vi "Get Magnet.vi"(6 "Axis":T1, 8 "error in (no error)":errorcluster, 11 "Instrument.Oxford1820 in":refnum<class "Instrument.Oxford1820.lvclass">) -> (0 "error out":errorcluster, 1 "Status":string, 2 "B Field (T)":dbl, 3 "Instrument.Oxford1820 out":refnum<class "Instrument.Oxford1820.lvclass">, 4 "Finished?":bool)   [LabVIEW 2019, in "Instrument.Oxford1820.lvclass"]
uses:
  Instrument.Oxford1820.lvclass
  <userlib>/LevyLab/Instrument Framework/Instrument Types/Cryostat/Typedefs/Magnet Axis--Enum.ctl
  4d514aa9-5884-4ec3-9942-9e0d55515c9c.vi
  Typedefs/Instrument.Oxford1820.Commands-enum.ctl
  c1f1fec1-7ced-457a-8a6a-e70d4f1fe444.vi
  <userlib>/LevyLab/LV-Data/LV-Data.PG/LV-Data.PGSQL.lvclass
  <userlib>/LevyLab/LV-Data/LV-Data.PG/API/Read Variable (string).vi
  <userlib>/LevyLab/LV-Data/LV-Data.PG/API/Read Variable (double).vi
  <userlib>/LevyLab/Instrument Framework/Instrument Types/Cryostat/Instrument.Cryostat.lvclass
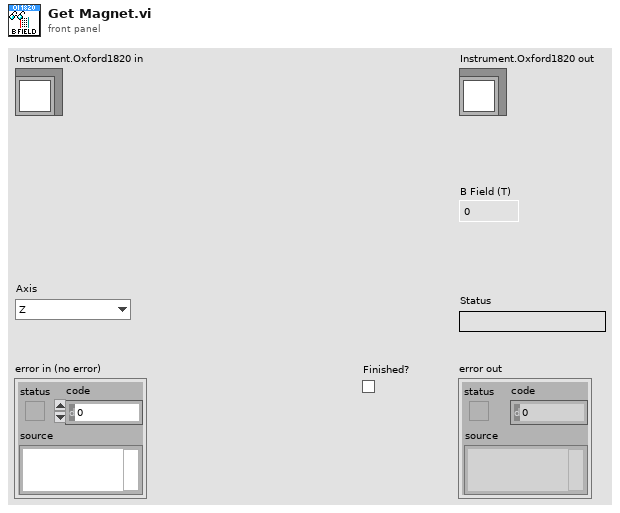
[diagram p1: front panel]
types:
  T1 = typedef "Instrument.Cryostat.lvclass/Magnet Axis--Enum.ctl" = enum16{"Z", "X", "Y"}
  T2 = typedef "Instrument.Oxford1820.lvclass/Instrument.Oxford1820.Commands-enum.ctl" = enum16{"setAction", "setTarget", "setSwitchHeat", "setLambda", "setFillMode", "setNeedleValve", "setMagnetField", "getStatus", "getTarget", "getSwitchHeat", "getPSUField", "setSequenceStatus", "getMagnetField"}
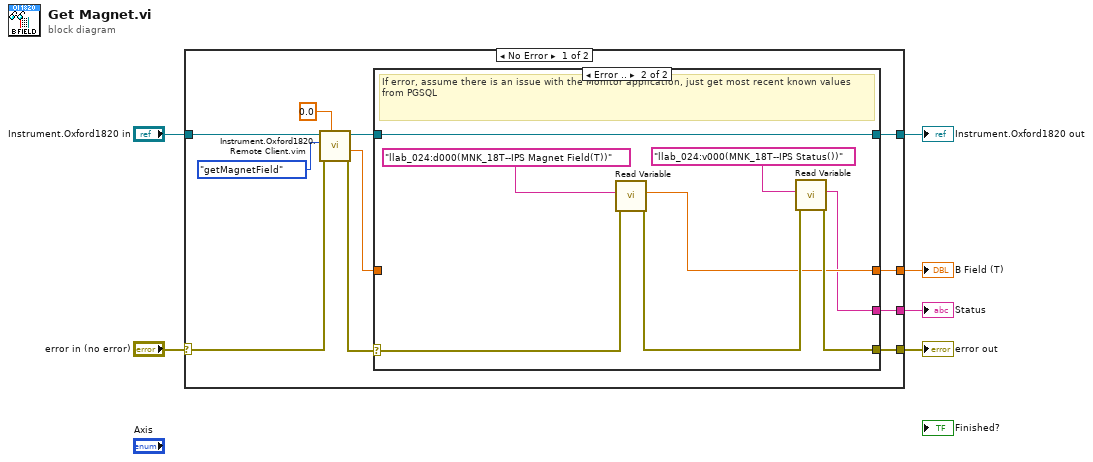
[diagram p0: block diagram]
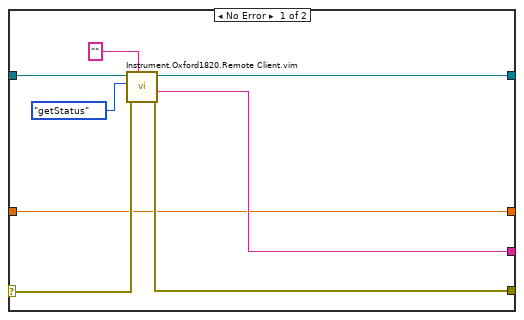
[diagram p2: hidden frame]
diagram:
  n1 = case shown="No Error" "error in (no error)" {
    selector: "error in (no error)" -> [w11 w35]
    tunnel: "Instrument.Oxford1820 in" -> [w12 w34]
    tunnel: [w8 w34] -> w5
    tunnel: [w17 _] -> w4
    tunnel: [w16 w35] -> w2
    tunnel: [w15 _] -> w1
    frame No Error {
      n2 = call "Instrument.Oxford1820.Remote Client.vim"("Data Out type"=0.0, "error in (no error)"=w11, "Commands"=Instrument.Oxford1820.Commands-enum."getMagnetField", "Instrument.1820 in"=w12) -> ("error out"=w10:errorcluster, "Data out"=w9:dbl, "Instrument.1820 out"=w13:refnum<class "Instrument.Oxford1820.lvclass">)  [unwired: 5 in]
      n3 = case shown="Error .." w10 {
        selector: w10 -> [w22 w31]
        tunnel: [w19 w27] -> w17
        tunnel: [w20 w30] -> w16
        tunnel: [w21 w26] -> w15
        tunnel: w13 -> [w25 w29]
        tunnel: w9 -> [w19 _]
        tunnel: [w23 w29] -> w8
        frame No Error {
          n4 = call "Instrument.Oxford1820.Remote Client.vim"("Data Out type"="", "error in (no error)"=w22, "Commands"=Instrument.Oxford1820.Commands-enum."getStatus", "Instrument.1820 in"=w25) -> ("error out"=w20:errorcluster, "Data out"=w21:string, "Instrument.1820 out"=w23:refnum<class "Instrument.Oxford1820.lvclass">)  [unwired: 5 in]
        }
        frame Error {
          # "If error, assume there is an issue with the Monitor application, just get most recent known values from PGSQL"
          n5 = call-poly <userlib>:"Read Variable.vi"("error in (no error)"=w31, "PG path"="llab_024:d000(MNK_18T--IPS Magnet Field(T))") -> ("error out"=w33:errorcluster, "Value"=w27:dbl)  [unwired: 4 in, 4 out]
          n6 = call-poly <userlib>:"Read Variable.vi"("error in (no error)"=w33, "PG path"="llab_024:v000(MNK_18T--IPS Status())") -> ("error out"=w30:errorcluster, "Value"=w26:string)  [unwired: 4 in, 4 out]
        }
      }
    }
    frame Error {
    }
  }
  "error out" <- w2
  "Instrument.Oxford1820 out" <- w5
  "B Field (T)" <- w4
  "Status" <- w1
